vi "HEWH Check Draws Remaining.vi"(8 "Error In":errorcluster, 10 "Station":string, 11 "DrawsLeft":i32[](array[numeric])) -> (0 "Error Out":errorcluster, 3 "Draws Remaining?":bool)   [LabVIEW 2019]
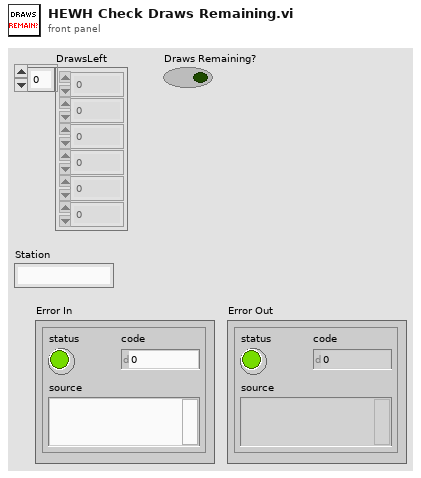
[diagram p1: front panel]
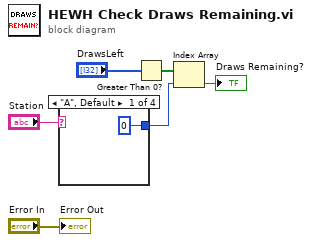
[diagram p0: block diagram]
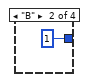
[diagram p2: hidden frame]
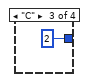
[diagram p3: hidden frame]
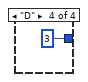
[diagram p4: hidden frame]
diagram:
  n1 = case shown="\"A\", Default" "Station" {
    tunnel: [0 ("index") 1 ("index") 2 ("index") 3 ("index")] -> w5
    frame "A", Default {
    }
    frame "B" {
    }
    frame "C" {
    }
    frame "D" {
    }
  }
  n2 = Greater Than 0?(x="DrawsLeft") -> (x > 0?=w2:bool[])
  n3 = Index Array(array=w2, index=w5) -> (element=→"Draws Remaining?":bool)
  "Error Out" <- "Error In"
